vi "prueba.vi"() -> ()   [LabVIEW 2015]
uses:
  <vilib>/userdefined/High Color/nirio_resource_hc.ctl
  <vilib>/FPGAPlugInAG/cRIO-9031/niLvFpga_Open_cRIO-9031.vi
  <vilib>/FPGAPlugInAG/cRIO-9031/niLvFpga_Run_cRIO-9031.vi
  <vilib>/Utility/error.llb/Error Cluster From Error Code.vi
  <vilib>/rvi/errors/niLvFpgaAdjustHostInterfaceError.vi
  <vilib>/FPGAPlugInAG/cRIO-9031/niLvFpga_Close_cRIO-9031.vi
  <vilib>/rvi/interface/nirviOpenFPGA/nirviOpenFPGA.xnode
  FPGA Bitfiles/W&RDArabia_FPGATarget_FPGA8a2wsBIdirec_yJvL9yuTbZw.lvbitx
  <vilib>/rvi/interface/nirviMethod/nirviMethod.xnode
  <vilib>/rvi/interface/nirviReadWriteControl/nirviReadWriteControl.xnode
  <vilib>/rvi/interface/nirviCloseFPGA/nirviCloseFPGA.xnode
  NiFpgaLv.dll
  <vilib>/FPGAPlugInAG/cRIO-9031/niLvFpga_ReadFifo_cRIO-9031.vi
  <vilib>/rvi/errors/niLvFpgaMergeErrorWithErrorCode.vi
panel:
  out "error out 2":errorcluster
  out "DC OK":bool
  out "Data":dbl[](array[numeric])
  out "error out":errorcluster
  out "Chassis Temperature":i16
  in  "stop":bool
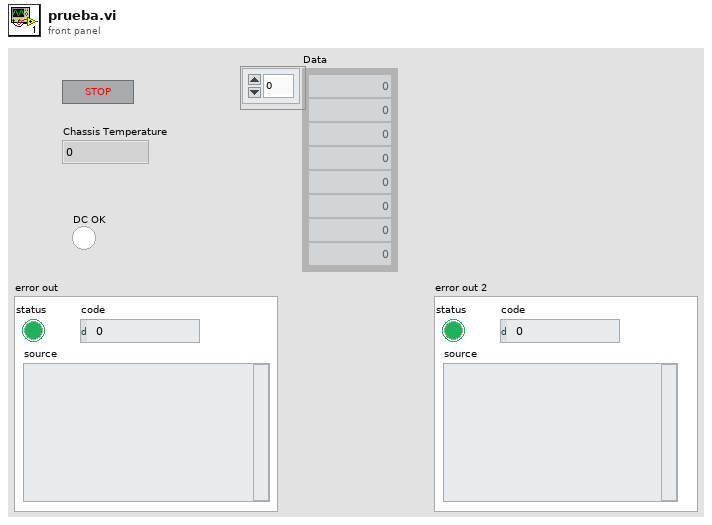
[diagram p1: front panel]
types:
  T1 = typedef "nirio_resource_hc.ctl" = tag
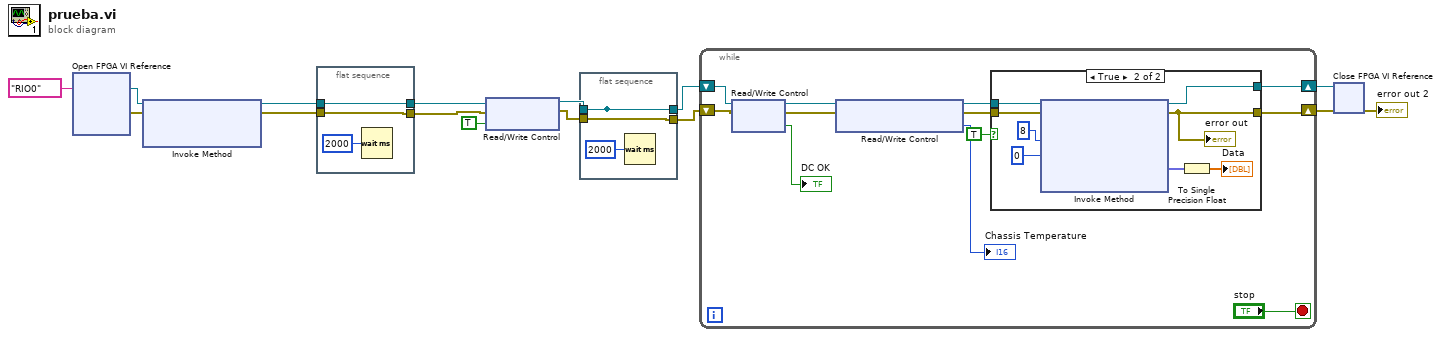
[diagram p0: block diagram]
diagram:
  n1 = xnode "Open FPGA VI Reference"("resource name"=T1 "RIO0") -> ("FPGA VI Reference Out"=w13:refnum<k20>, "error out"=w14:errorcluster)  [unwired: 1 in]
  n2 = xnode "Invoke Method"("FPGA VI Reference In"=w13, "error in"=w14) -> ("FPGA VI Reference Out"=w8:refnum<k20>, "error out"=w6:errorcluster)  [unwired: 1 in]
  n3 = flat-sequence {
    tunnel: w8 -> [w18]
    tunnel: [w18] -> w7
    tunnel: w6 -> [w17]
    tunnel: [w17] -> w5
    frame #0 {
      n4 = Wait (ms)(milliseconds to wait=u32 2000) -> ()  [unwired: 1 out]
    }
  }
  n5 = xnode "Read/Write Control"("FPGA VI Reference In"=w7, "error in"=w5, "Fotocélula"=TRUE) -> ("FPGA VI Reference Out"=w4:refnum<k20>, "error out"=w3:errorcluster)
  n6 = flat-sequence {
    tunnel: w4 -> [w19]
    tunnel: [w19] -> _
    tunnel: w3 -> [w21]
    tunnel: [w21] -> w2
    tunnel: [w19] -> w1
    frame #0 {
      n7 = Wait (ms)(milliseconds to wait=u32 2000) -> ()  [unwired: 1 out]
    }
  }
  n8 = while {
    shift-right: [w23] -> w10
    shift-left: w2 -> [w24]
    shift-right: [w27] -> w12
    shift-left: w1 -> [w25]
    stop <- "stop" stop-if-true
    n9 = xnode "Read/Write Control"("FPGA VI Reference In"=w25, "error in"=w24) -> ("FPGA VI Reference Out"=w32:refnum<k20>, "error out"=w31:errorcluster, "DC OK"=→"DC OK":bool)
    n10 = xnode "Read/Write Control"("FPGA VI Reference In"=w32, "error in"=w31) -> ("FPGA VI Reference Out"=w29:refnum<k20>, "error out"=w28:errorcluster, "Chassis Temperature"=→"Chassis Temperature":i16)
    n11 = case shown="True" TRUE {
      tunnel: w29 -> [w35 w42]
      tunnel: w28 -> [w34 w41]
      tunnel: [w35 w40] -> w27
      tunnel: [w34 w38] -> w23
      frame False {
      }
      frame True {
        n12 = xnode "Invoke Method"("FPGA VI Reference In"=w42, "error in"=w41, "Number of Elements"=u32 8, "Timeout (ms)"=0) -> ("FPGA VI Reference Out"=w40:refnum<k20>, "error out"=w38:errorcluster, "Data"=w37:fxp<+/-,24,4>[])  [unwired: 1 out]
        "error out" <- w38
        n13 = To Single Precision Float(number=w37) -> (single precision float=→"Data":sgl[])
      }
    }
  }
  n14 = xnode "Close FPGA VI Reference"("FPGA VI Reference In"=w12, "error in"=w10) -> ("error out"=→"error out 2":errorcluster)
